vi "ScanImg (SubVI).vi"(4 "pixel":i32, 6 "Channel index (0-23)":u8, 7 "Bias (V)":sgl, 8 "error in (no error)":errorcluster, 9 "Current":sgl, 10 "Img Speed":sgl, 11 "Application in":refnum<vi>) -> (0 "error out":errorcluster, 2 "Img":dbl[][](array[numeric]), 3 "Application out":refnum<vi>)   [LabVIEW 2014]
uses:
  <userlib>/Nanonis Prog Interface V5/Nanonis Prog Interface.lvlib
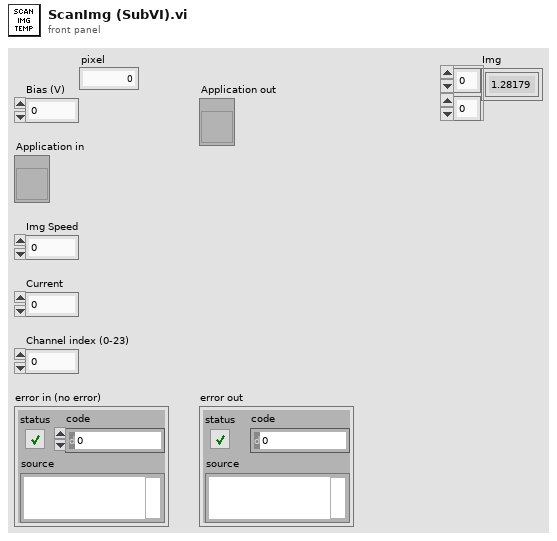
[diagram p1: front panel]
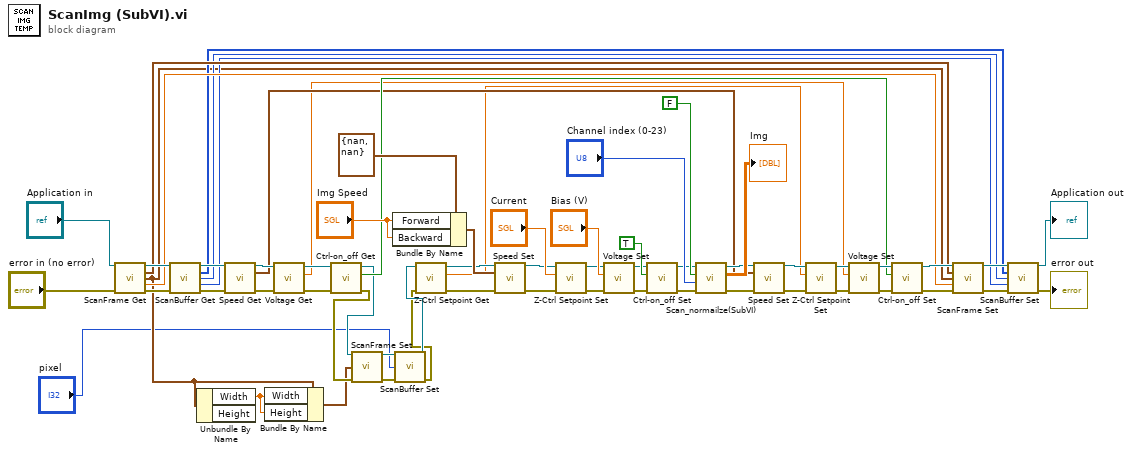
[diagram p0: block diagram]
diagram:
  n1 = call <userlib>:"ScanFrame Get.vi"("Application ref in"="Application in", "error in (no error)"="error in (no error)") -> ("Application ref out"=w25:refnum<vi>, "Center coordinates (m)"=w15:cluster{"Xc":sgl, "Yc":sgl}, "Size (m)"=w4:cluster{"Width":sgl, "Height":sgl}, "Angle (deg)"=w14:sgl, "error out"=w22:errorcluster)  [unwired: 9 in]
  n2 = call <userlib>:"ScanBuffer Get.vi"("Application ref in"=w25, "error in (no error)"=w22) -> ("Application ref out"=w24:refnum<vi>, "Channels indexes (0-23)"=w13:i32[], "Pixels/line"=w11:i32, "Lines"=w12:i32, "error out"=w23:errorcluster)  [unwired: 9 in]
  n3 = Unbundle By Name(w4) -> ("Width"=w2:sgl)  [unwired: 1 out]
  n4 = call <userlib>:"Speed Get.vi"("Application ref in"=w24, "error in (no error)"=w23) -> ("Application ref out"=w51:refnum<vi>, "Speed (m/s)"=w30:cluster{"Forward":sgl, "Backward":sgl}, "error out"=w50:errorcluster)  [unwired: 8 in, 3 out]
  n5 = Bundle By Name(cluster=w4, "Width"=w2, "Height"=w2) -> (w3:cluster{"Width":sgl, "Height":sgl})
  n6 = call <userlib>:"Voltage Get.vi"("error in (no error)"=w50, "Application ref in"=w51) -> ("error out"=w38:errorcluster, "Bias (V)"=w29:sgl, "Application ref out"=w39:refnum<vi>)  [unwired: 7 in]
  n7 = call <userlib>:"Ctrl-on_off Get.vi"("error in (no error)"=w38, "Application ref in"=w39) -> ("error out"=w7:errorcluster, "Z-Controller on/off status"=w31:bool, "Application ref out"=w10:refnum<vi>)  [unwired: 7 in]
  n8 = call <userlib>:"ScanFrame Set.vi"("Application ref in"=w10, "Size (m)"=w3, "error in (no error)"=w7) -> ("Application ref out"=w9:refnum<vi>, "error out"=w5:errorcluster)  [unwired: 11 in]
  n9 = Bundle By Name(cluster=cluster{"Forward":sgl, "Backward":sgl} {"Forward"=nan, "Backward"=nan} ("Speed (m/s)"), "Forward"="Img Speed", "Backward"="Img Speed") -> (w58:cluster{"Forward":sgl, "Backward":sgl})
  n10 = call <userlib>:"ScanBuffer Set.vi"("Application ref in"=w9, "Pixels"="pixel", "error in (no error)"=w5) -> ("Application ref out"=w8:refnum<vi>, "error out"=w6:errorcluster)  [unwired: 11 in]
  n11 = call <userlib>:"Z-Ctrl Setpoint Get.vi"("error in (no error)"=w6, "Application ref in"=w8) -> ("error out"=w42:errorcluster, "Z Controller setpoint"=w28:sgl, "Application ref out"=w43:refnum<vi>)  [unwired: 6 in]
  n12 = call <userlib>:"Speed Set.vi"("Application ref in"=w43, "Speed (m/s)"=w58, "error in (no error)"=w42) -> ("Application ref out"=w49:refnum<vi>, "error out"=w48:errorcluster)  [unwired: 11 in]
  n13 = call <userlib>:"Z-Ctrl Setpoint Set.vi"("error in (no error)"=w48, "Z Controller setpoint"="Current", "Application ref in"=w49) -> ("error out"=w46:errorcluster, "Application ref out"=w47:refnum<vi>)  [unwired: 7 in]
  n14 = call <userlib>:"Voltage Set.vi"("Error in (no error)"=w46, "Bias (V)"="Bias (V)", "Application ref in"=w47) -> ("Error out"=w45:errorcluster, "Application ref out"=w44:refnum<vi>)  [unwired: 7 in]
  n15 = call <userlib>:"Ctrl-on_off Set.vi"("error in (no error)"=w45, "Z Controller ON/OFF"=TRUE, "Application ref in"=w44) -> ("error out"=w54:errorcluster, "Application ref out"=w53:refnum<vi>)  [unwired: 7 in]
  n16 = call "Scan_normailze(SubVI).vi"("error in (no error)"=w54, "Channel index (0-23)"="Channel index (0-23)", "Normalization"=FALSE, "Application in"=w53) -> ("error out"=w32:errorcluster, "Array"=→"Img":dbl[][], "Application out"=w33:refnum<vi>)  [unwired: 5 in]
  n17 = call <userlib>:"Speed Set.vi"("Application ref in"=w33, "Speed (m/s)"=w30, "error in (no error)"=w32) -> ("Application ref out"=w35:refnum<vi>, "error out"=w41:errorcluster)  [unwired: 11 in]
  n18 = call <userlib>:"Z-Ctrl Setpoint Set.vi"("error in (no error)"=w41, "Z Controller setpoint"=w28, "Application ref in"=w35) -> ("error out"=w40:errorcluster, "Application ref out"=w36:refnum<vi>)  [unwired: 7 in]
  n19 = call <userlib>:"Voltage Set.vi"("Error in (no error)"=w40, "Bias (V)"=w29, "Application ref in"=w36) -> ("Error out"=w34:errorcluster, "Application ref out"=w37:refnum<vi>)  [unwired: 7 in]
  n20 = call <userlib>:"Ctrl-on_off Set.vi"("error in (no error)"=w34, "Z Controller ON/OFF"=w31, "Application ref in"=w37) -> ("error out"=w16:errorcluster, "Application ref out"=w21:refnum<vi>)  [unwired: 7 in]
  n21 = call <userlib>:"ScanFrame Set.vi"("Application ref in"=w21, "Center coordinates (m)"=w15, "Size (m)"=w4, "Angle (deg)"=w14, "error in (no error)"=w16) -> ("Application ref out"=w20:refnum<vi>, "error out"=w17:errorcluster)  [unwired: 9 in]
  n22 = call <userlib>:"ScanBuffer Set.vi"("Application ref in"=w20, "Channels indexes (0-23)"=w13, "Pixels"=w11, "Lines"=w12, "error in (no error)"=w17) -> ("Application ref out"=→"Application out":refnum<vi>, "error out"=→"error out":errorcluster)  [unwired: 9 in]
